vi "GUI.vi"(8 "ErrorIn":errorcluster, 11 "QueuesIn":T1) -> (0 "ErrorOut":errorcluster={"status"=TRUE, "code"=1, "source"="Dequeue Element in commandQueues.vi->GUI.vi->main.vi"}, 3 "QueuesOut":T1)   [LabVIEW 2019]
uses:
  utilities/Queues.ctl
  GUIVIs/GUIOutput.ctl
  MobileAnalyzer/mainVIs/analyzeAccelerationDataVIs/AnalyzedVibrationsData.ctl
  MobileAnalyzer/mainVIs/analyzeAccelerationDataVIs/AccelerationDataFrames.ctl
  MobileAnalyzer/mainVIs/analyzeAccelerationDataVIs/calculateFaultIndicatorsVIs/FaultDetections.ctl
  MobileAnalyzer/mainVIs/analyzeAccelerationDataVIs/calculateFaultIndicatorsVIs/ParameterFaultDetection.ctl
  MobileAnalyzer/mainVIs/analyzeAccelerationDataVIs/calculateFaultIndicatorsVIs/FaultParameter.ctl
  MobileAnalyzer/mainVIs/analyzeAccelerationDataVIs/calculateFaultIndicatorsVIs/FrequencyFaultDetection.ctl
  MobileAnalyzer/mainVIs/analyzeAccelerationDataVIs/calculateFaultIndicatorsVIs/OrdersFaultDetection.ctl
  masterVIs/Command.ctl
  MobileAnalyzer/mainVIs/TDMSmanagerVIs/TDMSAnalyzerData.ctl
  MobileAnalyzer/mainVIs/TDMSmanagerVIs/TDMSAnalyzerDataType.ctl
  saveAccelerationTimeDataToTDMSVIs/DataToSave.ctl
  masterVIs/Thread.ctl
  MobileAnalyzer/mainVIs/utilities/FGVAction.ctl
panel:
  out "Prędkość obrotowa [obr/min]":dbl
  out "Rzędy":string[](array[string])
  in  "Adres IP":string="172.22.11.2"
  in  "Clear charts":bool
  out "Pasma":string[](array[string])
  out "Wsp. szczytu":bool
  in  "Download analysis data":bool
  out "RMS":bool
  out "Kurtoza":bool
  in  "AnalyzerSettings":bool
  in  "Tab Plots":T2(tab)
  out "Przyspieszenia drgań w czasie":waveform(dbl)[](graph)
  out "FFT - Amplitudy":cluster{"f0":dbl, "df":dbl, "real part":dbl[]}[](graph) caption="FFT-AmplitudeAcceleration"
  out "FFT - Fazy":T3(graph)
  out "Syg. tachometru":waveform(dbl)(graph)
  out "Analiza rzędów":T3(graph)
  out "Kurtoza":dbl[][](graph)
  out "RMS":dbl[][](graph)
  out "Wsp. szczytu":dbl[][](graph)
  out "Pasma":dbl[][](graph)
  out "Wskazane pasma":dbl[][](graph)
  in  "Open data file":bool
  in  "Connect":bool
  in  "Start":bool
  in  "Stop":bool
  in  "Restart":bool
  out "Akwizycja danych":bool
  out "Analiza danych":bool
  in  "Exit":bool
  out "Polączono":bool
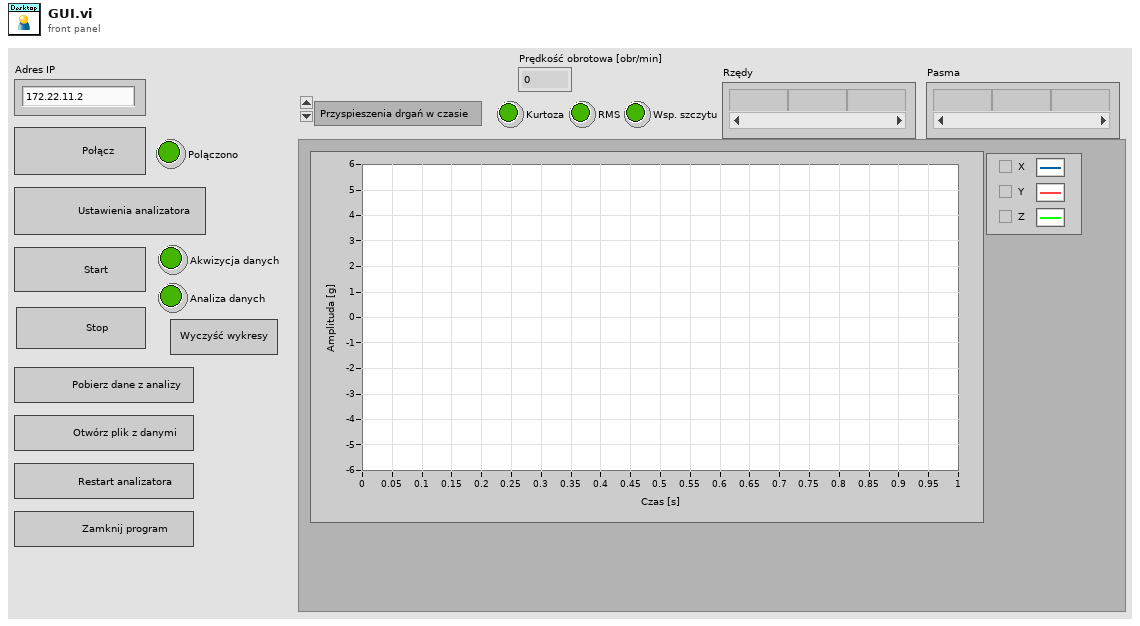
[diagram p1: front panel]
types:
  T1 = typedef "Queues.ctl" = cluster{"GUIOutput":refnum<queue>, "AnalyzedVibrationsData":refnum<queue>, "Command":refnum<queue>, "TDMSAnalyzerData":refnum<queue>, "DataToSave":refnum<queue>}
  T2 = enum32{"Przyspieszenia drgań w czasie", "FFT - amplitudy", "FFT - fazy", "Sygnał tachometru", "Analiza rzędów", "Kurtoza", "RMS", "Wsp. szczytu", "Pasma", "Wskazane rzędy"}
  T3 = cluster{"f0":dbl, "df":dbl, "imaginary part":dbl[]}[]
  T4 = typedef "Command.ctl" = enum16{"None", "Connect", "Start", "Stop", "RestartAnalyzer", "Exit", "OpenDataFile", "CanBegin", "FileToSaveSettings", "AnalyzerSettings", "DownloadDataDialog", "DownloadData", "DeleteData"}
  T5 = typedef "FGVAction.ctl" = enum16{"Read", "Write"}
  T6 = typedef "Thread.ctl" = enum16{"GUI", "communicateWithAnalyzer", "saveDataToTDMS"}
  T7 = typedef "DesktopAppSettings.ctl" = cluster{"MobileAnalyzer IP":string, "Network Stream Timeout Code":i32, "Endpoint Destroyed Code":i32, "Save to file?":bool, "All threads":T6[], "Connected":bool, "AnalysisSettings":T8}
  T8 = typedef "AnalysisSettings.ctl" = cluster{"Fault Thresholds":T9, "Analysis series name":string, "Save data analysis?":bool, "Band size":i32, "OrderAnalysis?":bool, "Accelerometer":T11, "fs [Hz]":dbl}
  T9 = typedef "Thresholds.ctl" = cluster{"Parameters labels":T10[], "Parameters thresholds":dbl[], "Freqs and thresholds":dbl[][], "Orders and thresholds":dbl[][]}
  T10 = typedef "FaultParameter.ctl" = enum16{"Kurtosis", "RMS", "Crest factor"}
  T11 = typedef "Accelerometer.ctl" = enum16{"None", "MPU6050", "MMA7351"}
  T12 = typedef "GUIOutput.ctl" = cluster{"Aquiring data":bool, "AnalyzerError":errorcluster, "FIFO overflow":bool, "Analyzing data":bool, "Connected":bool}
  T13 = typedef "AnalyzedVibrationsData.ctl" = cluster{"AccelerationDataFrames":T14, "Fault detections":T15, "Order Power Spectra":cluster{"order 0":dbl, "delta order":dbl, "magnitude":dbl[]}[], "Tacho signal":waveform(dbl), "Rotational speed [RPM]":dbl}
  T14 = typedef "AccelerationDataFrames.ctl" = cluster{"AccelerationData":waveform(dbl)[], "Amplitudes":cluster{"f0":dbl, "df":dbl, "real part":dbl[]}[], "Phases":cluster{"f0":dbl, "df":dbl, "imaginary part":dbl[]}[]}
  T15 = typedef "FaultDetections.ctl" = cluster{"Parameters fault detection":T16[], "Frequencies fault detection":T17[], "Orders fault detection":T18[]}
  T16 = typedef "ParameterFaultDetection.ctl" = cluster{"Axes Values":dbl[], "Axes Fault Detection":bool[], "Parameter Label":T10}
  T17 = typedef "FrequencyFaultDetection.ctl" = cluster{"Axes Values":dbl[], "Axes Fault Detection":bool[], "Frequency":dbl}
  T18 = typedef "OrdersFaultDetection.ctl" = cluster{"Order":dbl, "Axes Fault Detection":bool[], "Axes Values":dbl[]}
  T19 = cluster{"order 0":dbl, "delta order":dbl, "magnitude":dbl[]}[]
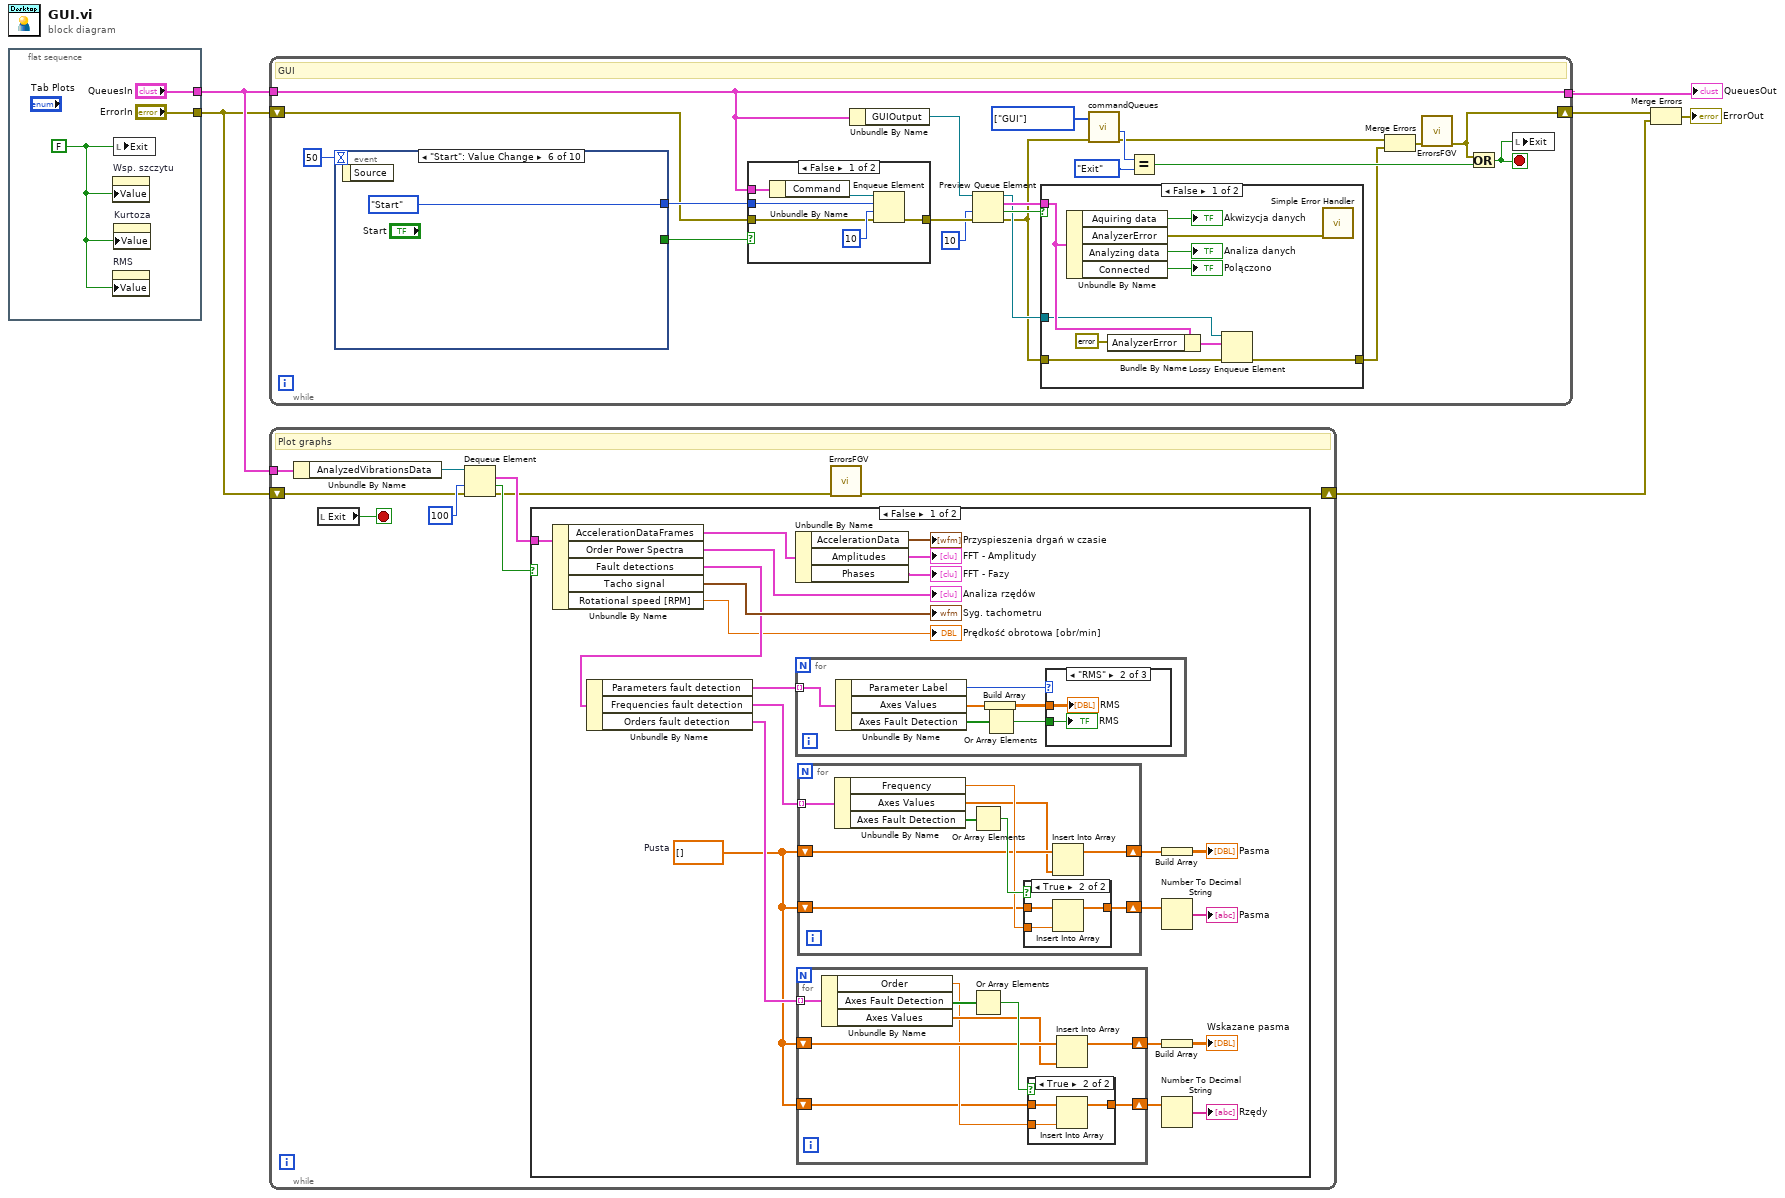
[diagram p0: block diagram]
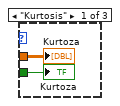
[diagram p4: hidden frame]
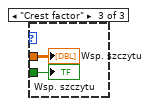
[diagram p5: hidden frame]
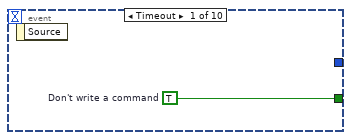
[diagram p9: hidden frame]
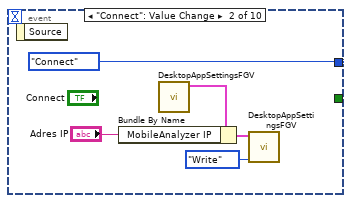
[diagram p10: hidden frame]
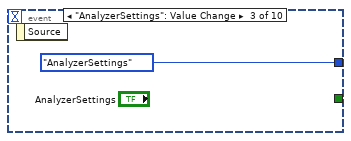
[diagram p11: hidden frame]
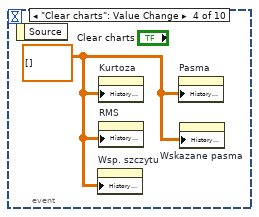
[diagram p12: hidden frame]
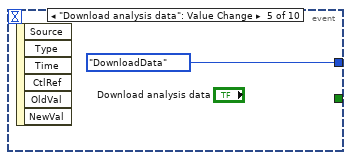
[diagram p13: hidden frame]
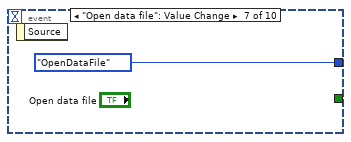
[diagram p14: hidden frame]
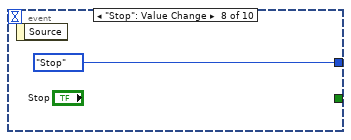
[diagram p15: hidden frame]
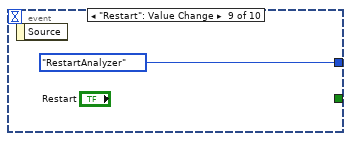
[diagram p16: hidden frame]
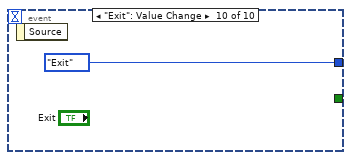
[diagram p17: hidden frame]
diagram:
  n1 = flat-sequence {
    tunnel: ["QueuesIn"] -> w6
    tunnel: ["ErrorIn"] -> w5
    frame #0 {
      w7 = FALSE ("Exit")
      n2 = property on="Wsp. szczytu" class="Bool (strict)"("Value"=w7) -> ()  [unwired: 2 in, 2 out]
      n3 = property on="RMS" class="Bool (strict)"("Value"=w7) -> ()  [unwired: 2 in, 2 out]
      n4 = local write "Exit"(w7) -> ()
      n5 = property on="Kurtoza" class="Bool (strict)"("Value"=w7) -> ()  [unwired: 2 in, 2 out]
    }
  }
  n6 = while {
    tunnel: w6 -> [w27]
    tunnel: [w27] -> w1
    shift-right: [w14] -> w4
    shift-left: w5 -> [w20]
    stop <- w21 stop-if-true
    w17 = T6[] [enum."GUI"] items=["GUI", "communicateWithAnalyzer", "saveDataToTDMS"] ("Threads")
    # "GUI"
    n7 = event shown="[5] \"Start\": Value Change" {
      selector: _ -> [_ _ _ _ _ _ _ _ _ _]
      dyn-events: _ -> [_ _ _ _ _ _ _ _ _ _]
      timeout: 50 -> [_ _ _ _ _ _ _ _ _ _]
      tunnel: [w49 _ _ _ _ _ _ _ _ _] -> w29
      tunnel: [_ Command."Connect" ("Command") Command."AnalyzerSettings" ("Command") _ Command."DownloadData" ("Command") Command."Start" ("Command") Command."OpenDataFile" ("Command") Command."Stop" ("Command") Command."RestartAnalyzer" ("Command") Command."Exit" ("Command")] -> w28
      event Timeout {
        w49 = TRUE  # Don't write a command
        n8 = event-data() -> ()  [unwired: 1 in, 1 out]
      }
      event "Connect": Value Change {
        n9 = event-data() -> ()  [unwired: 1 in, 1 out]
        n10 = call "DesktopAppSettingsFGV.vi"() -> ("DesktopAppSettingsOut"=w53:T7)  [unwired: 11 in]
        n11 = Bundle By Name(cluster=w53, "MobileAnalyzer IP"="Adres IP") -> (w51:T7)
        n12 = call "DesktopAppSettingsFGV.vi"("FGVAction (Read)"=FGVAction."Write", "DesktopAppSettingsIn"=w51) -> ()  [unwired: 9 in, 1 out]
      }
      event "AnalyzerSettings": Value Change {
        n13 = event-data() -> ()  [unwired: 1 in, 1 out]
      }
      event "Clear charts": Value Change {
        w56 = dbl[][] [] ("History Data")
        n14 = event-data() -> ()  [unwired: 1 in, 1 out]
        n15 = property on="Wsp. szczytu" class="WFChart (strict)"("History Data"=w56) -> ()  [unwired: 2 in, 2 out]
        n16 = property on="Kurtoza" class="WFChart (strict)"("History Data"=w56) -> ()  [unwired: 2 in, 2 out]
        n17 = property on="RMS" class="WFChart (strict)"("History Data"=w56) -> ()  [unwired: 2 in, 2 out]
        n18 = property on="Pasma" class="WFChart (strict)"("History Data"=w56) -> ()  [unwired: 2 in, 2 out]
        n19 = property on="Wskazane pasma" class="WFChart (strict)"("History Data"=w56) -> ()  [unwired: 2 in, 2 out]
      }
      event "Download analysis data": Value Change {
        n20 = event-data() -> ()  [unwired: 1 in, 6 out]
      }
      event "Start": Value Change {
        n21 = event-data() -> ()  [unwired: 1 in, 1 out]
      }
      event "Open data file": Value Change {
        n22 = event-data() -> ()  [unwired: 1 in, 1 out]
      }
      event "Stop": Value Change {
        n23 = event-data() -> ()  [unwired: 1 in, 1 out]
      }
      event "Restart": Value Change {
        n24 = event-data() -> ()  [unwired: 1 in, 1 out]
      }
      event "Exit": Value Change {
        n25 = event-data() -> ()  [unwired: 1 in, 1 out]
      }
    }
    n26 = case shown="False" w29 {
      tunnel: w28 -> [w45 _]
      tunnel: w27 -> [w44 _]
      tunnel: w20 -> [w43 w48]
      tunnel: [w42 w48] -> w25
      frame False {
        n27 = Unbundle By Name(w44) -> ("Command"=w47:refnum<queue>)
        n28 = Enqueue Element(queue=w47, element=w45, timeout in ms (-1)=10, error in (no error)=w43) -> (error out=w42:errorcluster)  [unwired: 2 out]
      }
      frame True {
      }
    }
    n29 = Unbundle By Name(w27) -> ("GUIOutput"=w26:refnum<queue>)
    n30 = Preview Queue Element(queue=w26, timeout in ms (-1)=10, error in (no error)=w25) -> (queue out=w13:refnum<queue>, element=w22:T12, timed out?=w23:bool, error out=w12:errorcluster)
    n31 = case shown="False" w23 {
      tunnel: w22 -> [w36 _]
      tunnel: w13 -> [w33 _]
      tunnel: w12 -> [w32 w41]
      tunnel: [w31 w41] -> w10
      frame False {
        n32 = Unbundle By Name(w36) -> ("Aquiring data"=→"Akwizycja danych":bool, "AnalyzerError"=w37:errorcluster, "Analyzing data"=→"Analiza danych":bool, "Connected"=→"Polączono":bool)
        n33 = Bundle By Name(cluster=w36, "AnalyzerError"=errorcluster {"status"=FALSE, "code"=0, "source"=""}) -> (w34:T12)
        n34 = Lossy Enqueue Element(queue=w33, element=w34, error in (no error)=w32) -> (error out=w31:errorcluster)  [unwired: 3 out]
        n35 = call <vilib>:"Simple Error Handler.vi"("error in (no error)"=w37) -> ()  [unwired: 4 in, 5 out]
      }
      frame True {
      }
    }
    n36 = call "commandQueues.vi"("ErrorIn"=w12, "Threads"=w17) -> ("ErrorOut"=w15:errorcluster, "CommandOut"=w19:T4)  [unwired: 8 in]
    n37 = Equal?(x=w19, y=Command."Exit") -> (x = y?=w16:bool)
    n38 = Merge Errors(w15, w10) -> (w11:errorcluster)
    n39 = call "ErrorsFGV.vi"("CriticalErrorIn"=w11) -> ("CriticalErrorOut"=w14:errorcluster)  [unwired: 7 in, 3 out]
    n40 = Or(x=w14, y=w16) -> (x .or. y?=w21:bool)
    n41 = local write "Exit"(w21) -> ()
  }
  "QueuesOut" <- w1
  n42 = while {
    tunnel: w6 -> [w64]
    shift-right: [w65] -> w2
    shift-left: w5 -> [w68]
    stop <- w67 stop-if-true
    # "Plot graphs"
    n43 = Unbundle By Name(w64) -> ("AnalyzedVibrationsData"=w63:refnum<queue>)
    n44 = local read "Exit"() -> (w67:bool)
    n45 = Dequeue Element(queue=w63, timeout in ms (-1)=100, error in (no error)=w68) -> (element=w71:T13, timed out?=w70:bool, error out=w66:errorcluster)  [unwired: 1 out]
    n46 = case shown="False" w70 {
      tunnel: w71 -> [w92 _]
      frame False {
        w78 = dbl[] []  # Pusta
        # "Plots"
        n47 = Unbundle By Name(w92) -> ("AccelerationDataFrames"=w91:T14, "Order Power Spectra"=→"Analiza rzędów":T19, "Fault detections"=w73:T15, "Tacho signal"=→"Syg. tachometru":waveform(dbl), "Rotational speed [RPM]"=→"Prędkość obrotowa [obr/min]":dbl)
        n48 = Unbundle By Name(w73) -> ("Parameters fault detection"=w87:T16[], "Frequencies fault detection"=w86:T17[], "Orders fault detection"=w79:T18[])
        n49 = Unbundle By Name(w91) -> ("AccelerationData"=→"Przyspieszenia drgań w czasie":waveform(dbl)[], "Amplitudes"=→"FFT - Amplitudy":cluster{"f0":dbl, "df":dbl, "real part":dbl[]}[], "Phases"=→"FFT - Fazy":T3)
        n50 = for {
          tunnel: w87 -> [w120] mode=indexing
          n51 = Unbundle By Name(w120) -> ("Parameter Label"=w119:T10, "Axes Values"=w121:dbl[], "Axes Fault Detection"=w123:bool[])
          n52 = Build Array(w121) -> (w122:dbl[][])
          n53 = Or Array Elements(Boolean array=w123) -> (logical OR=w124:bool)
          n54 = case shown="\"RMS\"" w119 {
            tunnel: w124 -> [w126 w128 w129]
            tunnel: w122 -> [w125 w127 w130]
            frame "Kurtosis" {
              "Kurtoza" <- w125
              "Kurtoza" <- w126
            }
            frame "RMS" {
              "RMS" <- w128
              "RMS" <- w127
            }
            frame "Crest factor" {
              "Wsp. szczytu" <- w130
              "Wsp. szczytu" <- w129
            }
          }
        }
        n55 = for {
          tunnel: w79 -> [w101] mode=indexing
          shift-right: [w97] -> w75
          shift-left: w78 -> [w98]
          shift-right: [w93] -> w77
          shift-left: w78 -> [w94]
          n56 = Unbundle By Name(w101) -> ("Order"=w95:dbl, "Axes Fault Detection"=w99:bool[], "Axes Values"=w96:dbl[])
          n57 = Or Array Elements(Boolean array=w99) -> (logical OR=w100:bool)
          n58 = case shown="True" w100 {
            tunnel: [w102 w105] -> w93
            tunnel: w95 -> [_ w104]
            tunnel: w94 -> [w102 w103]
            frame False {
            }
            frame True {
              n59 = Insert Into Array(array=w103, new element=w104) -> (w105:dbl[])  [unwired: 1 in]
            }
          }
          n60 = Insert Into Array(array=w98, new element=w96) -> (w97:dbl[])  [unwired: 1 in]
        }
        n61 = for {
          tunnel: w86 -> [w114] mode=indexing
          shift-right: [w109] -> w85
          shift-left: w78 -> [w110]
          shift-right: [w106] -> w83
          shift-left: w78 -> [w108]
          n62 = Unbundle By Name(w114) -> ("Frequency"=w111:dbl, "Axes Values"=w107:dbl[], "Axes Fault Detection"=w113:bool[])
          n63 = Or Array Elements(Boolean array=w113) -> (logical OR=w112:bool)
          n64 = case shown="True" w112 {
            tunnel: w111 -> [_ w118]
            tunnel: w110 -> [w115 w117]
            tunnel: [w115 w116] -> w109
            frame False {
            }
            frame True {
              n65 = Insert Into Array(array=w117, new element=w118) -> (w116:dbl[])  [unwired: 1 in]
            }
          }
          n66 = Insert Into Array(array=w108, new element=w107) -> (w106:dbl[])  [unwired: 1 in]
        }
        n67 = Build Array(w83) -> (→"Pasma":dbl[][])
        n68 = Number To Decimal String(number=w85) -> (decimal integer string=→"Pasma":string[])  [unwired: 1 in]
        n69 = Build Array(w75) -> (→"Wskazane pasma":dbl[][])
        n70 = Number To Decimal String(number=w77) -> (decimal integer string=→"Rzędy":string[])  [unwired: 1 in]
      }
      frame True {
      }
    }
    n71 = call "ErrorsFGV.vi"("CriticalErrorIn"=w66) -> ("CriticalErrorOut"=w65:errorcluster)  [unwired: 7 in, 3 out]
  }
  n72 = Merge Errors(w4, w2) -> (→"ErrorOut":errorcluster)
